vi "acqComponentsInit_v1.vi"(1 "405 nm filter":T3(ring), 2 "488 nm filter":T3(ring)=enum."525/50 [FITC]", 3 "561 nm filter":T3(ring)=enum."605/70 [Cy3]", 4 "642 nm filter":T3(ring)=enum."665/LP [Cy5]", 6 "405 nm (aq)":bool=TRUE, 8 "488 nm (aq)":bool=TRUE, 10 "561 nm (aq)":bool=TRUE, 12 "642 nm (aq)":bool=TRUE) -> (15 "Initialized filters":T2(array[ring])=[enum."460/36 [DAPI]", enum."525/50 [FITC]", enum."605/70 [Cy3]", enum."665/LP [Cy5]"], 16 "initializedLasers":T1(array[cluster]), 17 "correctCompInit?":bool)   [LabVIEW 2015]
panel:
  in  "LSFM_3 lasers":T1(array[cluster])=[{"Component ID"="405nm", "COM Port"="COM14", "Type "=enum."omicronLuxX", "init"=1}, {"Component ID"="488nm", "COM Port"="COM4", "Type "=enum."omicronLuxX", "init"=1}, {"Component ID"="561nm", "COM Port"="COM27", "Type "=enum."coherentObis", "init"=1}, {"Component ID"="642nm", "COM Port"="COM12", "Type "=enum."omicronLuxX", "init"=1}]
  out "Correct lasers init?":i32=1
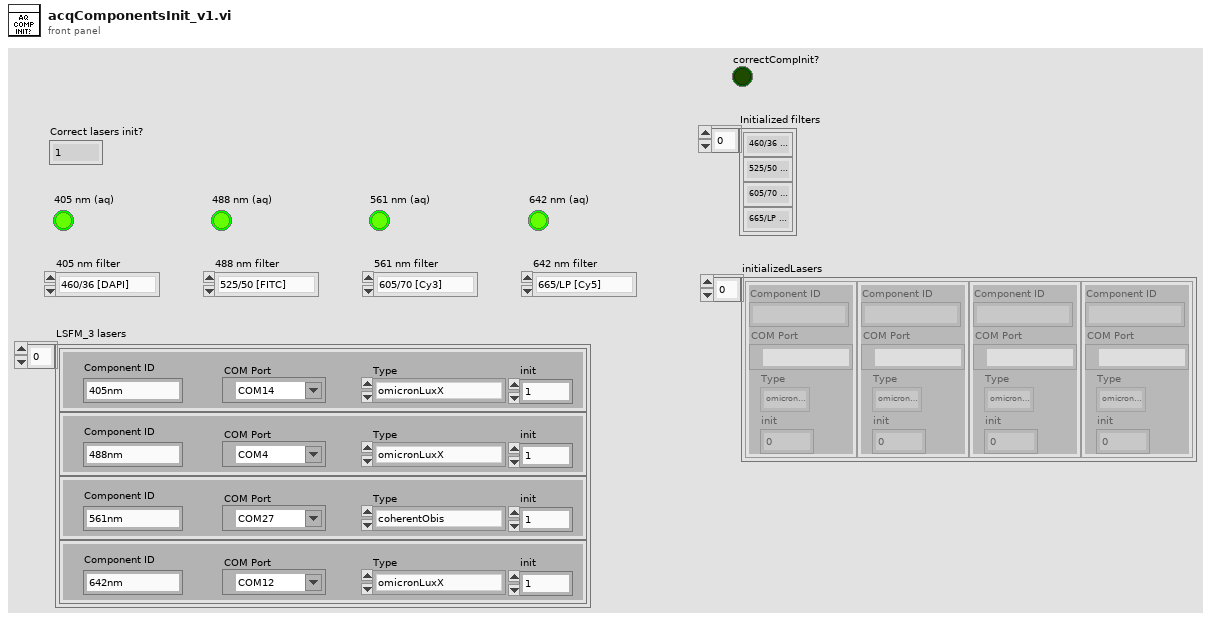
[diagram p1: front panel]
types:
  T1 = cluster{"Component ID":string, "COM Port":refnum<visa-resource-name>, "Type ":enum16{"omicronLuxX", "coherentObis"}, "init":i16}[]
  T2 = enum16{"460/36 [DAPI]", "525/50 [FITC]", "605/70 [Cy3]", "665/LP [Cy5]", "Empty-1", "Empty-2"}[]
  T3 = enum16{"460/36 [DAPI]", "525/50 [FITC]", "605/70 [Cy3]", "665/LP [Cy5]", "Empty-1", "Empty-2"}
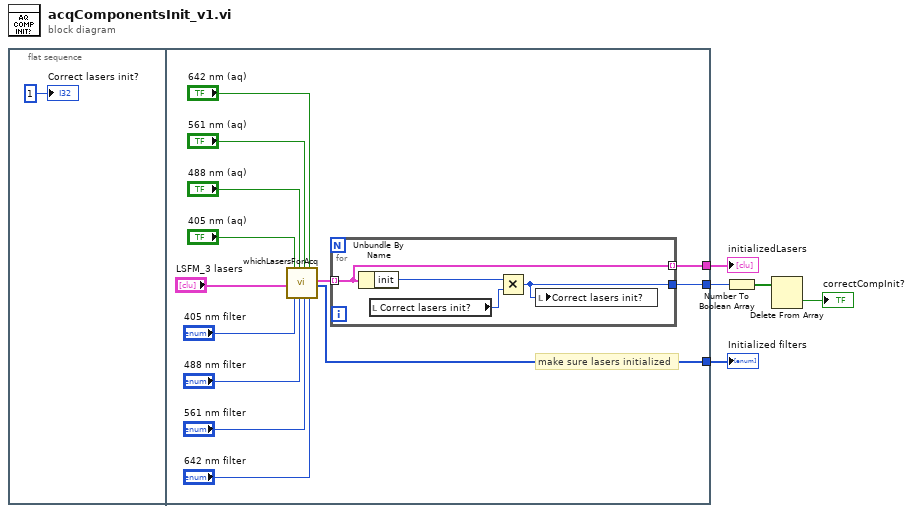
[diagram p0: block diagram]
diagram:
  n1 = flat-sequence {
    tunnel: [w9] -> w3
    tunnel: [w8] -> w5
    tunnel: [w10] -> w4
    frame #0 {
      "Correct lasers init?" <- 1 ("Correct lasers init?")
    }
    frame #1 {
      # "make sure lasers initialized"
      n2 = call "whichLasersForAcq.vi"("LSFM_3 lasers"="LSFM_3 lasers", "405 nm (aq)"="405 nm (aq)", "405 nm filter"="405 nm filter", "488 nm (aq)"="488 nm (aq)", "488 nm filter"="488 nm filter", "561 nm (aq)"="561 nm (aq)", "561 nm filter"="561 nm filter", "642 nm (aq)"="642 nm (aq)", "642 nm filter"="642 nm filter") -> ("Initialized lasers"=w19:T1, "Array 2"=w10:T2)  [unwired: 9 in]
      n3 = for {
        tunnel: w19 -> [w20] mode=indexing
        tunnel: [w21] -> w9
        tunnel: [w20] -> w8 mode=indexing
        n4 = Unbundle By Name(w20) -> ("init"=w23:i16)
        n5 = local read "Correct lasers init?"() -> (w22:i32)
        n6 = Multiply(x=w23, y=w22) -> (x*y=w21:i32)
        n7 = local write "Correct lasers init?"(w21) -> ()
      }
    }
  }
  n8 = Number To Boolean Array(number=w3) -> (Boolean array=w2:bool[])
  n9 = Delete From Array(array=w2) -> (deleted portion=→"correctCompInit?":bool)  [unwired: 2 in, 1 out]
  "initializedLasers" <- w5
  "Initialized filters" <- w4
